vi "TEMOCR-Open IPC.vi"() -> (8 "IPC":T1)   [LabVIEW 2015]
uses:
  Typedefs/TEMOCR-IPC.ctl
  Typedefs/TEMOCR-Parameters.ctl
  Typedefs/TEMOCR-Probe.ctl
  Typedefs/TEMOCR-Elicitor.ctl
  Human Studies/SFM Frontend/LV Source/Typedefs/HSTS-Transducer.ctl
  Typedefs/TEMOCR-Sequence.ctl
  Typedefs/TEMOCR-Analysis.ctl
  CFTS Main Panel SubVIs/CFTS-Experiment State.ctl
  Typedefs/TEMOCR-Sequence Step.ctl
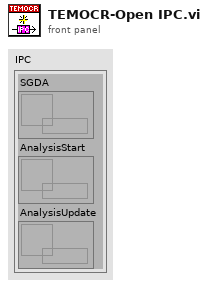
[diagram p1: front panel]
types:
  T1 = typedef "TEMOCR-IPC.ctl" = cluster{"SGDA":refnum<queue>, "AnalysisStart":refnum<queue>, "AnalysisUpdate":refnum<queue>}
  T2 = typedef "TEMOCR-Sequence Step.ctl" = cluster{"Rep":i32, "Seq":i32, "Phase":i32}
  T3 = typedef "TEMOCR-Parameters.ctl" = cluster{"Probe":T4, "Elicitor":T5, "Sequence":T7, "Analysis":T8, "Repeats":i32, "Fs (Hz)":dbl, "Cycles":i32, "save raw":bool}
  T4 = typedef "TEMOCR-Probe.ctl" = cluster{"Ear":enum16{"Right", "Left"}, "Stimulus":enum16{"Click", "Chirp"}, "Duration (us)":dbl, "Nclick":i32, "ICI (ms)":dbl, "Level":dbl}
  T5 = typedef "TEMOCR-Elicitor.ctl" = cluster{"Onset (s)":dbl, "Offset (s)":dbl, "Ramp (ms)":dbl, "Transducer":T6}
  T6 = typedef "HSTS-Transducer.ctl" = enum16{"Insert", "TDH-39", "HD300", "ER-10X"}
  T7 = typedef "TEMOCR-Sequence.ctl" = cluster{"Start":dbl, "Stop":dbl, "Step":dbl}
  T8 = typedef "TEMOCR-Analysis.ctl" = cluster{"Tmin (ms)":dbl, "Tmax (ms)":dbl, "Fmin (Hz)":dbl, "Fmax (Hz)":dbl, "Window":enum16{"None", "Hanning", "Hamming"}, "Fhp (Hz)":dbl, "Flp (Hz)":dbl, "Gain (dB)":dbl}
  T9 = typedef "CFTS-Experiment State.ctl" = cluster{"Experimenter":string, "Number":u32, "Right":string, "Left":string, "Data Folder":path, "State File":path, "Version Info":string, "End Exposure Time":dbl, "Exposure Duration":string, "Run #":cluster{"CAP":i16, "ABR":i16, "DP":i16, "VsEP":i16, "MeasSeq":i16, "SubSeq":i16, "SFOAE":i16}}
  T10 = cluster{"queue out":refnum<queue>, "queue out":refnum<queue>, "queue out":refnum<queue>}
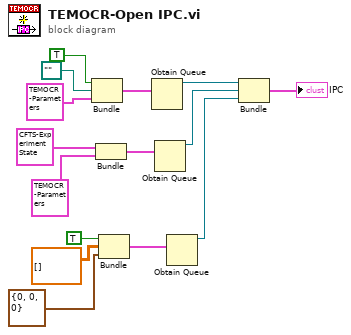
[diagram p0: block diagram]
diagram:
  n1 = Bundle(TRUE, path "", "Params"=T3 {"Probe"={"Ear"=enum."Right", "Stimulus"=enum."Click", "Duration (us)"=0.0, "Nclick"=0, "ICI (ms)"=0.0, "Level"=0.0}, "Elicitor"={"Onset (s)"=0.0, "Offset (s)"=0.0, "Ramp (ms)"=0.0, "Transducer"=enum."Insert"}, "Sequence"={"Start"=0.0, "Stop"=0.0, "Step"=0.0}, "Analysis"={"Tmin (ms)"=0.0, "Tmax (ms)"=0.0, "Fmin (Hz)"=0.0, "Fmax (Hz)"=0.0, "Window"=enum."None", "Fhp (Hz)"=0.0, "Flp (Hz)"=0.0, "Gain (dB)"=0.0}, "Repeats"=0, "Fs (Hz)"=0.0, "Cycles"=0, "save raw"=FALSE}) -> (w14:cluster{bool, path, "Params":T3})  [unwired: 1 in]
  n2 = Bundle("Expt State"=T9 {"Experimenter"="", "Number"=0, "Right"="", "Left"="", "Data Folder"=path "", "State File"=path "", "Version Info"="", "End Exposure Time"=0.0, "Exposure Duration"="", "Run #"={"CAP"=0, "ABR"=0, "DP"=0, "VsEP"=0, "MeasSeq"=0, "SubSeq"=0, "SFOAE"=0}}, "Params"=T3 {"Probe"={"Ear"=enum."Right", "Stimulus"=enum."Click", "Duration (us)"=0.0, "Nclick"=0, "ICI (ms)"=0.0, "Level"=0.0}, "Elicitor"={"Onset (s)"=0.0, "Offset (s)"=0.0, "Ramp (ms)"=0.0, "Transducer"=enum."Insert"}, "Sequence"={"Start"=0.0, "Stop"=0.0, "Step"=0.0}, "Analysis"={"Tmin (ms)"=0.0, "Tmax (ms)"=0.0, "Fmin (Hz)"=0.0, "Fmax (Hz)"=0.0, "Window"=enum."None", "Fhp (Hz)"=0.0, "Flp (Hz)"=0.0, "Gain (dB)"=0.0}, "Repeats"=0, "Fs (Hz)"=0.0, "Cycles"=0, "save raw"=FALSE}) -> (w8:cluster{"Expt State":T9, "Params":T3})  [unwired: 1 in]
  n3 = Bundle(TRUE, dbl[][] [], "Sequence"=T2 {"Rep"=0, "Seq"=0, "Phase"=0}) -> (w11:cluster{bool, dbl[][], "Sequence":T2})  [unwired: 1 in]
  n4 = Obtain Queue(element data type=w14) -> (queue out=w7:refnum<queue>)  [unwired: 4 in, 2 out]
  n5 = Obtain Queue(element data type=w8) -> (queue out=w6:refnum<queue>)  [unwired: 4 in, 2 out]
  n6 = Obtain Queue(element data type=w11) -> (queue out=w5:refnum<queue>)  [unwired: 4 in, 2 out]
  n7 = Bundle("queue out"=w7, "queue out"=w6, "queue out"=w5) -> (→"IPC":T10)  [unwired: 1 in]
